vi "Write to Digital Line Continuousy.vi"() -> ()   [LabVIEW 2020]
uses:
  <vilib>/DAQmx/write.llb/DAQmx Write (Digital Bool 1Line 1Point).vi
  <vilib>/DAQmx/create/channels.llb/DAQmx Create Channel (DO-Digital Output).vi
  <vilib>/DAQmx/miscellaneous.llb/DAQmx Fill In Error Info.vi
panel:
  in  "stop":bool
  in  "milliseconds to wait":u64
  in  "DAQmx Physical Channel":tag
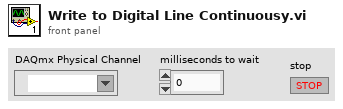
[diagram p1: front panel]
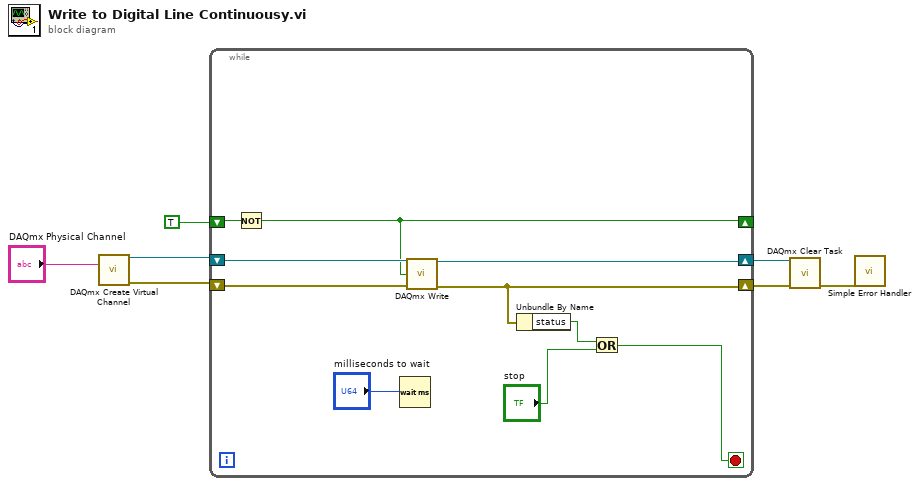
[diagram p0: block diagram]
diagram:
  n1 = call-poly <vilib>:"DAQmx Create Virtual Channel.vi"("lines"="DAQmx Physical Channel") -> ("task out"=w6:refnum<k21>, "error out"=w5:errorcluster)  [unwired: 13 in]
  n2 = while {
    shift-right: [w15] -> w3
    shift-left: w6 -> [w16]
    shift-right: [w11] -> w2
    shift-left: w5 -> [w14]
    shift-right: [w12] -> _
    shift-left: TRUE -> [w17]
    stop <- w8 stop-if-true
    n3 = Not(x=w17) -> (.not. x?=w12:bool)
    n4 = Wait (ms)(milliseconds to wait="milliseconds to wait") -> ()  [unwired: 1 out]
    n5 = call-poly <vilib>:"DAQmx Write.vi"("task/channels in"=w16, "data"=w12, "error in"=w14) -> ("task out"=w15:refnum<k21>, "error out"=w11:errorcluster)  [unwired: 10 in, 1 out]
    n6 = Unbundle By Name(w11) -> ("status"=w9:bool)
    n7 = Or(x=w9, y="stop") -> (x .or. y?=w8:bool)
  }
  n8 = call <vilib>:"DAQmx Clear Task.vi"("task in"=w3, "error in"=w2) -> ("error out"=w1:errorcluster)  [unwired: 13 in]
  n9 = call <vilib>:"Simple Error Handler.vi"("error in (no error)"=w1) -> ()  [unwired: 4 in, 5 out]
